vi "Timeout.vi"(2 "Done with Task?":bool, 3 "Timeout (ms)":u32) -> (0 "Timed Out?":bool)   [LabVIEW 2013]
panel:
  # "A vi for Dectecting if a Wait in a State Machine has Been Waiting \ntoo Long and Needs to Resend its Command"
  # "due to the issue with deciding when to initialize this, it looks like a FG inside..."
  # "...but it isn't so don't be decieved..."
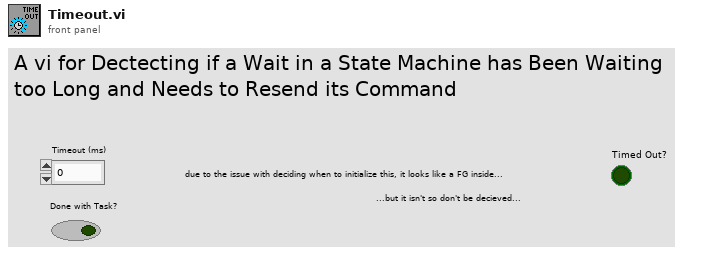
[diagram p1: front panel]
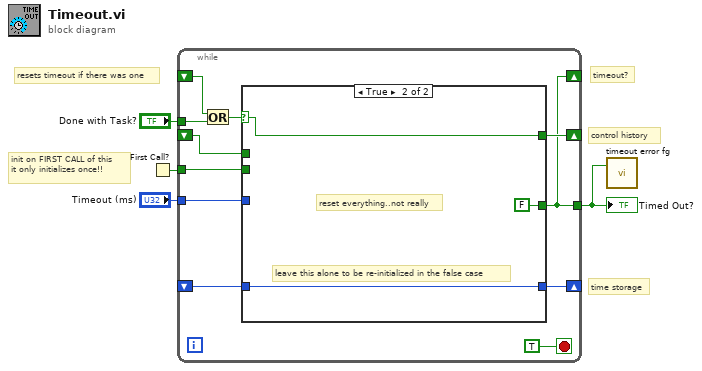
[diagram p0: block diagram]
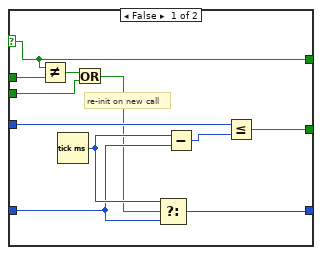
[diagram p2: hidden frame]
diagram:
  # "resets timeout if there was one"
  # "timeout?"
  # "init on FIRST CALL of this\nit only initializes once!!"
  # "control history"
  # "time storage"
  n1 = First Call?() -> (First Call?: T/F=w2:bool)
  n2 = while {
    tunnel: "Timeout (ms)" -> [w12]
    shift-right: [w14] -> _
    shift-left: _ -> [w13]
    tunnel: [w8] -> w1
    shift-right: [w11] -> _
    shift-left: _ -> [w10]
    tunnel: "Done with Task?" -> [w7]
    tunnel: w2 -> [w9]
    shift-right: [w8] -> _
    shift-left: _ -> [w6]
    stop <- TRUE stop-if-true
    n3 = Or(x=w6, y=w7) -> (x .or. y?=w5:bool)
    n4 = case shown="True" w5 {
      selector: w5 -> [w20 w28]
      tunnel: [w24 w27] -> w14
      tunnel: w13 -> [w23 w27]
      tunnel: w12 -> [w22 _]
      tunnel: [w21 FALSE] -> w8
      tunnel: [w20 w28] -> w11
      tunnel: w10 -> [w19 _]
      tunnel: w9 -> [w16 _]
      frame False {
        # "re-init on new call"
        n5 = Not Equal?(x=w20, y=w19) -> (x != y?=w18:bool)
        n6 = Tick Count (ms)() -> (millisecond timer value=w26:u32)
        n7 = Or(x=w18, y=w16) -> (x .or. y?=w17:bool)
        n8 = Select(t=w26, s=w17, f=w23) -> (s? t:f=w24:u32)
        n9 = Subtract(x=w26, y=w23) -> (x-y=w25:u32)
        n10 = Less Or Equal?(x=w22, y=w25) -> (x <= y?=w21:bool)
      }
      frame True {
        # "leave this alone to be re-initialized in the false case"
        # "reset everything..not really"
      }
    }
  }
  "Timed Out?" <- w1
  n11 = call "timeout error fg.vi"("Timeout Error?"=w1) -> ()  [unwired: 1 in, 2 out]
